vi "FPGA Main.vi"() -> ()   [LabVIEW 2020]
uses:
  src/FPGA/Public/Type Defs/Communication References.ctl
  src/FPGA/Public/Type Defs/BCI-1553 References.ctl
  <vilib>/rvi/Emulation/niFpgaGetClockAttributes.vi
  <vilib>/rvi/Emulation/niFpgaSctlEmulationGetInTimedLoop.vi
  <vilib>/rvi/Emulation/niFpgaEmulationReportErrorSimple.vi
  <vilib>/rvi/Emulation/niFpgaProcessEmulError.vi
  <vilib>/rvi/Emulation/niFpgaCriticalErrorInLSC.vi
  src/FPGA/BCI-1553 RT Interface.lvlib
panel:
  in  "Stop":bool
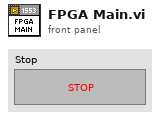
[diagram p1: front panel]
types:
  T1 = typedef "BCI-1553 RT Interface.lvlib/BCI-1553 References.ctl" = cluster{"BCI-1553 Device 0":refnum<k21>, "BCI-1553 Device 1":refnum<k21>, "BCI-1553 Device 2":refnum<k21>, "BCI-1553 Device 3":refnum<k21>, "BCI-1553 Device 4":refnum<k21>, "BCI-1553 Device 5":refnum<k21>, "BCI-1553 Device 6":refnum<k21>, "BCI-1553 Device 7":refnum<k21>}
  T2 = typedef "BCI-1553 RT Interface.lvlib/Communication References.ctl" = cluster{"BCI-1553-RSP":refnum<k21>, "BCI-1553-CMD":refnum<k21>}
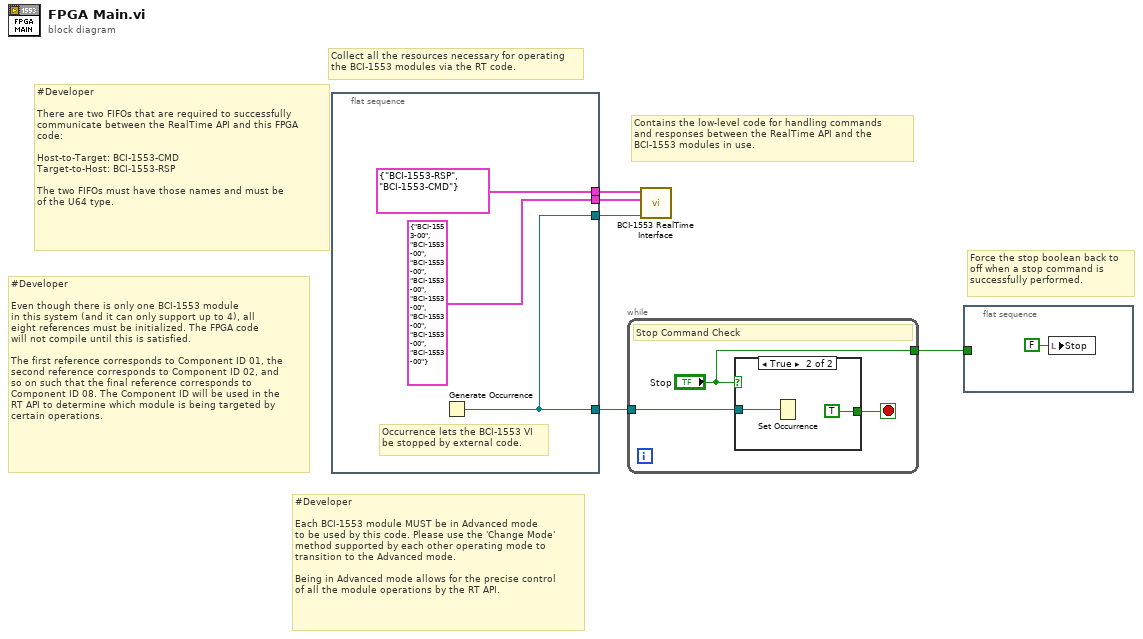
[diagram p0: block diagram]
diagram:
  # "#Developer\n\nEach BCI-1553 module MUST be in Advanced mode\nto be used by this code. Please use the 'Change Mode'\nmethod supported by each other operating mode to\ntransition to the Advanced mode.\n\nBeing in Advanced mode allows for the precise control\nof all the module operations by the RT API."
  # "Contains the low-level code for handling commands\nand responses between the RealTime API and the \nBCI-1553 modules in use."
  # "#Developer\n\nEven though there is only one BCI-1553 module\nin this system (and it can only support up to 4), all\neight references must be initialized. The FPGA code\nwill not compile until this is satisfied.\n\nThe first reference corresponds to Component ID 01, the\nsecond reference corresponds to Component ID 02, and\nso on such that the final reference corresponds to\nComponent ID 08. The Component ID will be used in the\nRT API to determine which module is being targeted by\ncertain operations."
  # "#Developer\n\nThere are two FIFOs that are required to successfully\ncommunicate between the RealTime API and this FPGA\ncode:\n\nHost-to-Target: BCI-1553-CMD\nTarget-to-Host: BCI-1553-RSP\n\nThe two FIFOs must have those names and must be\nof the U64 type."
  # "Collect all the resources necessary for operating\nthe BCI-1553 modules via the RT code."
  # "Force the stop boolean back to\noff when a stop command is\nsuccessfully performed."
  n1 = flat-sequence {
    tunnel: [T2 {"BCI-1553-RSP"="BCI-1553-RSP", "BCI-1553-CMD"="BCI-1553-CMD"} ("Communication References")] -> w5
    tunnel: [T1 {"BCI-1553 Device 0"="BCI-1553-00", "BCI-1553 Device 1"="BCI-1553-00", "BCI-1553 Device 2"="BCI-1553-00", "BCI-1553 Device 3"="BCI-1553-00", "BCI-1553 Device 4"="BCI-1553-00", "BCI-1553 Device 5"="BCI-1553-00", "BCI-1553 Device 6"="BCI-1553-00", "BCI-1553 Device 7"="BCI-1553-00"} ("BCI-1553 References")] -> w4
    tunnel: [w6] -> w3
    tunnel: [w6] -> w2
    frame #0 {
      # "Occurrence lets the BCI-1553 VI\nbe stopped by external code."
      n2 = Generate Occurrence() -> (w6:refnum<k4>)
    }
  }
  n3 = while {
    tunnel: w2 -> [w11]
    tunnel: ["Stop"] -> w1
    stop <- w10 stop-if-true
    # "Stop Command Check"
    n4 = case shown="True" "Stop" {
      tunnel: w11 -> [_ w13]
      tunnel: [_ TRUE] -> w10
      frame False {
      }
      frame True {
        n5 = Set Occurrence(w13) -> ()
      }
    }
  }
  n6 = call "BCI-1553 RealTime Interface.vi"("Stop Occurrence"=w3, "BCI-1553 References"=w4, "Communication References"=w5) -> ()  [unwired: 9 in]
  n7 = flat-sequence {
    tunnel: w1 -> [_]
    frame #0 {
      n8 = local write "Stop"(FALSE ("Stop")) -> ()
    }
  }
